vi "Write Nested Viewable Enqueuers.vi"(8 "error in (no error)":errorcluster, 9 "Viewable Names (optional)":string[](array[string]), 10 "Nested Viewable Enqueuers":refnum<class "Message Enqueuer.lvclass">[](array[class]), 11 "BoundViewManager In":refnum<class "BoundViewManager.lvclass">) -> (0 "error out":errorcluster, 3 "BoundViewManager Out":refnum<class "BoundViewManager.lvclass">)   [LabVIEW 2017, in "BoundViewManager.lvlib" / "BoundViewManager.lvclass"]
doc: "<License>\nCopyright © 2017 Composed Systems, LLC | All rights reserved\nwww.composed.io\n\nAuthor: Ethan Stern <ethan.stern@composed.io>\n\nThis software is provided \"AS IS\" WITHOUT WARRANTIES, either express or implied, AND IS FOR EDUCATIONAL PURPOSES ONLY.\n</License>"
uses:
  BoundViewManager.lvclass
  <vilib>/ActorFramework/Message Enqueuer/Message Enqueuer.lvclass
  BoundViewManager.lvclass/BoundViewManager.ctl
  <vilib>/Composed Systems/Current Value Table/CurrentValueTable.lvclass
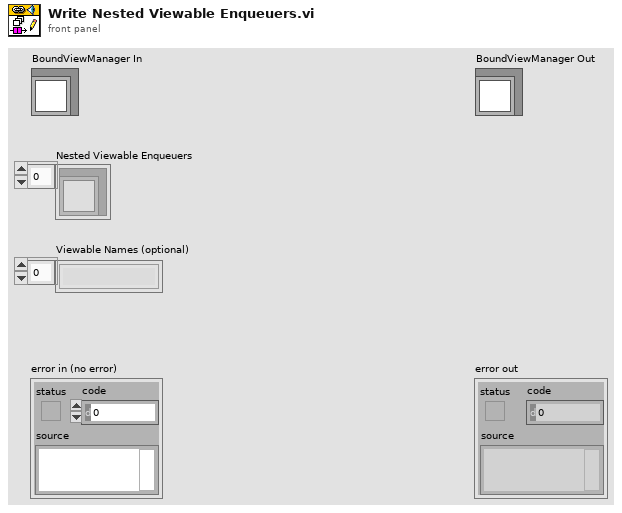
[diagram p1: front panel]
types:
  T1 = typedef "CurrentValueTable.lvlib/CurrentValueTable.lvclass/CurrentValueTable Reference.ctl" = refnum<data-value>
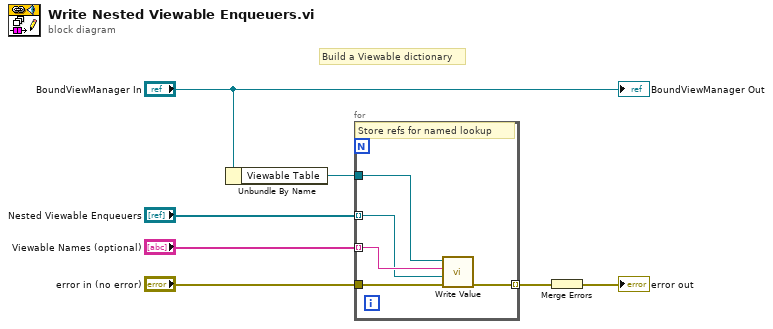
[diagram p0: block diagram]
diagram:
  # "Build a Viewable dictionary"
  n1 = Unbundle By Name("BoundViewManager In") -> ("Viewable Table"=w3:T1)
  n2 = for {
    tunnel: w3 -> [w12]
    tunnel: "Viewable Names (optional)" -> [w11] mode=indexing
    tunnel: "Nested Viewable Enqueuers" -> [w10] mode=indexing
    tunnel: [w9] -> w6 mode=indexing
    tunnel: "error in (no error)" -> [w8]
    # "Store refs for named lookup"
    n3 = call <vilib>:"Write Value.vi"("error in (no error)"=w8, "Value"=w10, "Data Name (Use Value Name)"=w11, "Current Value Table"=w12) -> ("error out"=w9:errorcluster)  [unwired: 6 in, 1 out]
  }
  n4 = Merge Errors(w6) -> (→"error out":errorcluster)
  "BoundViewManager Out" <- "BoundViewManager In"
